vi "ReadData_9229.vi"(8 "error in":errorcluster, 11 "Module Config Selector":i16) -> (0 "error out":errorcluster, 1 "Number Of Pulses":u32, 2 "OversampleClk Ticks":u32, 3 "Data Array":sgl[](array[numeric]) format="%.2f")   [LabVIEW 2017, in "VDMS_VibAPI_8.lvlib"]
uses:
  <vilib>/addons/InsightCM/Devices/Shared/Cms/Fpga/AcquisitionFpgaTach/source/subVIs/VibAPI_8/VDMS_VibAPI_8.lvlib
  <vilib>/rvi/eio/common/nirviEmuTemplateMethod_errors.vi
  <vilib>/rvi/Memory/Memory_Emulation/nirvimemoryFastEmulation.vi
  <vilib>/rvi/Memory/Memory_Emulation/nirvimemoryEmulation.vi
  <vilib>/rvi/Emulation/niFpgaEmulationIsFPGAContextNoSignature.vi
  <vilib>/rvi/DataTransferAndStorage/Container/Common/niFpgaContainerGetUniqueNameForEmu.vi
  <vilib>/rvi/Emulation/niFpgaProcessEmulError.vi
  <vilib>/rvi/Emulation/niFpgaSctlEmulationGetInTimedLoop.vi
  <vilib>/rvi/errors/nirviReportUnexpectedCaseInternalError (U32).vi
  <vilib>/eio/EIONode/EIONode.xnode
  <vilib>/rvi/DataTransferAndStorage/Container/XNode/niFpgaContainer.xnode
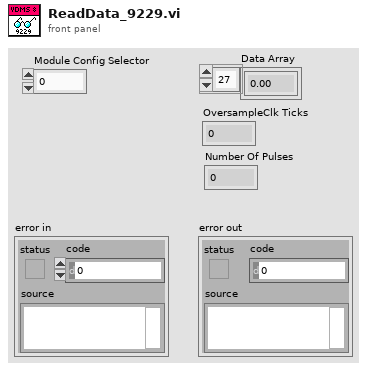
[diagram p1: front panel]
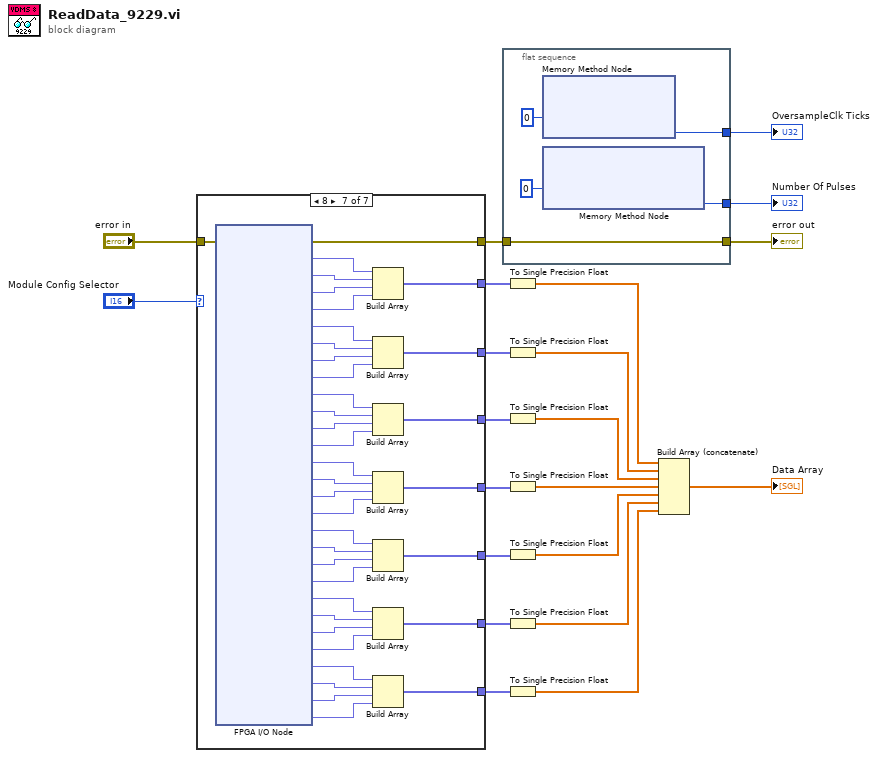
[diagram p0: block diagram]
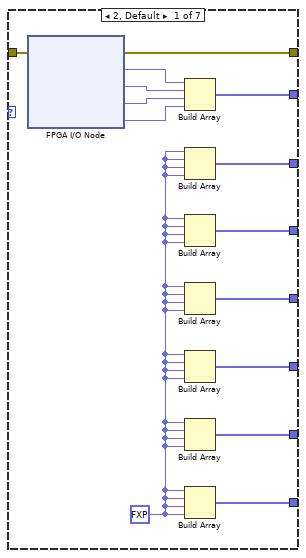
[diagram p2: hidden frame]
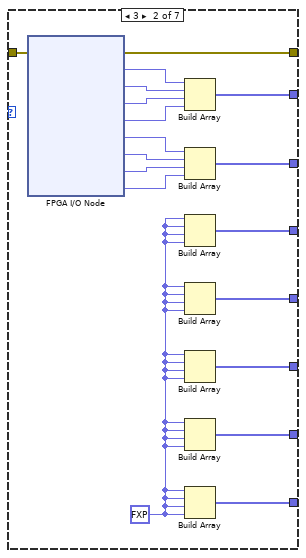
[diagram p3: hidden frame]
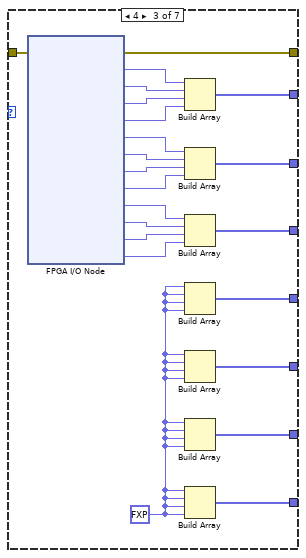
[diagram p4: hidden frame]
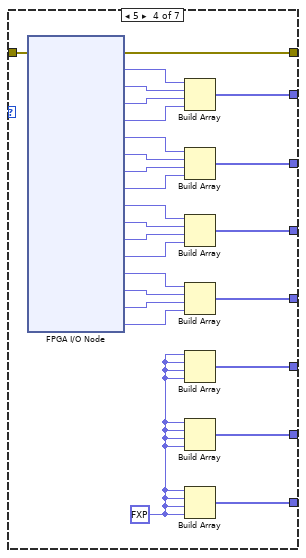
[diagram p5: hidden frame]
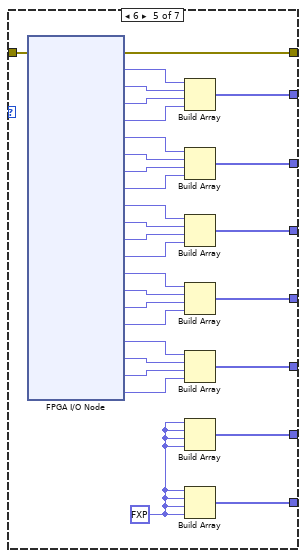
[diagram p6: hidden frame]
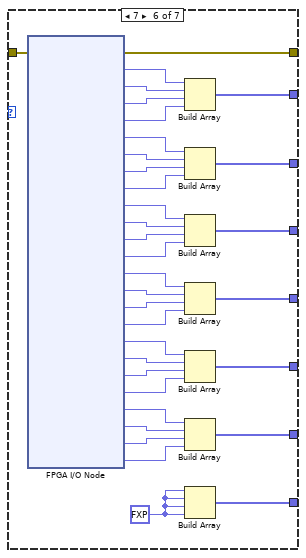
[diagram p7: hidden frame]
diagram:
  n1 = case shown="8" "Module Config Selector" {
    tunnel: "error in" -> [w35 w53 w75 w101 w131 w165 w202]
    tunnel: [w34 w52 w74 w100 w130 w164 w201] -> w21
    tunnel: [w33 w51 w73 w99 w129 w163 w200] -> w17
    tunnel: [w32 w50 w72 w98 w128 w162 w199] -> w15
    tunnel: [w31 w49 w71 w97 w127 w161 w198] -> w12
    tunnel: [w30 w48 w70 w96 w126 w160 w197] -> w10
    tunnel: [w29 w47 w69 w95 w125 w159 w196] -> w8
    tunnel: [w28 w46 w68 w94 w124 w158 w195] -> w6
    tunnel: [w27 w45 w67 w93 w123 w157 w194] -> w4
    frame 2, Default {
      w22 = fxp<+/-,24,7> 0.0 ("Mod1/AI2")
      n2 = xnode "FPGA I/O Node"("error in"=w35) -> ("error out"=w34:errorcluster, "Mod2/AI0"=w25:fxp<+/-,24,7>, "Mod2/AI1"=w26:fxp<+/-,24,7>, "Mod2/AI2"=w24:fxp<+/-,24,7>, "Mod2/AI3"=w23:fxp<+/-,24,7>)  [unwired: 4 in, 4 out]
      n3 = Build Array(w25, w26, w24, w23) -> (w33:fxp<+/-,24,7>[])
      n4 = Build Array(w22, w22, w22, w22) -> (w32:fxp<+/-,24,7>[])
      n5 = Build Array(w22, w22, w22, w22) -> (w31:fxp<+/-,24,7>[])
      n6 = Build Array(w22, w22, w22, w22) -> (w30:fxp<+/-,24,7>[])
      n7 = Build Array(w22, w22, w22, w22) -> (w29:fxp<+/-,24,7>[])
      n8 = Build Array(w22, w22, w22, w22) -> (w28:fxp<+/-,24,7>[])
      n9 = Build Array(w22, w22, w22, w22) -> (w27:fxp<+/-,24,7>[])
    }
    frame 3 {
      w36 = fxp<+/-,24,7> 0.0 ("Mod1/AI2")
      n10 = xnode "FPGA I/O Node"("error in"=w53) -> ("error out"=w52:errorcluster, "Mod2/AI0"=w41:fxp<+/-,24,7>, "Mod2/AI1"=w42:fxp<+/-,24,7>, "Mod2/AI2"=w40:fxp<+/-,24,7>, "Mod2/AI3"=w38:fxp<+/-,24,7>, "Mod3/AI0"=w39:fxp<+/-,24,7>, "Mod3/AI1"=w43:fxp<+/-,24,7>, "Mod3/AI2"=w44:fxp<+/-,24,7>, "Mod3/AI3"=w37:fxp<+/-,24,7>)  [unwired: 8 in, 8 out]
      n11 = Build Array(w41, w42, w40, w38) -> (w51:fxp<+/-,24,7>[])
      n12 = Build Array(w39, w43, w44, w37) -> (w50:fxp<+/-,24,7>[])
      n13 = Build Array(w36, w36, w36, w36) -> (w49:fxp<+/-,24,7>[])
      n14 = Build Array(w36, w36, w36, w36) -> (w48:fxp<+/-,24,7>[])
      n15 = Build Array(w36, w36, w36, w36) -> (w47:fxp<+/-,24,7>[])
      n16 = Build Array(w36, w36, w36, w36) -> (w46:fxp<+/-,24,7>[])
      n17 = Build Array(w36, w36, w36, w36) -> (w45:fxp<+/-,24,7>[])
    }
    frame 4 {
      w54 = fxp<+/-,24,7> 0.0 ("Mod1/AI2")
      n18 = xnode "FPGA I/O Node"("error in"=w75) -> ("error out"=w74:errorcluster, "Mod2/AI0"=w60:fxp<+/-,24,7>, "Mod2/AI1"=w61:fxp<+/-,24,7>, "Mod2/AI2"=w59:fxp<+/-,24,7>, "Mod2/AI3"=w57:fxp<+/-,24,7>, "Mod3/AI0"=w58:fxp<+/-,24,7>, "Mod3/AI1"=w62:fxp<+/-,24,7>, "Mod3/AI2"=w63:fxp<+/-,24,7>, "Mod3/AI3"=w56:fxp<+/-,24,7>, "Mod4/AI0"=w64:fxp<+/-,24,7>, "Mod4/AI1"=w65:fxp<+/-,24,7>, "Mod4/AI2"=w66:fxp<+/-,24,7>, "Mod4/AI3"=w55:fxp<+/-,24,7>)  [unwired: 12 in, 12 out]
      n19 = Build Array(w60, w61, w59, w57) -> (w73:fxp<+/-,24,7>[])
      n20 = Build Array(w58, w62, w63, w56) -> (w72:fxp<+/-,24,7>[])
      n21 = Build Array(w64, w65, w66, w55) -> (w71:fxp<+/-,24,7>[])
      n22 = Build Array(w54, w54, w54, w54) -> (w70:fxp<+/-,24,7>[])
      n23 = Build Array(w54, w54, w54, w54) -> (w69:fxp<+/-,24,7>[])
      n24 = Build Array(w54, w54, w54, w54) -> (w68:fxp<+/-,24,7>[])
      n25 = Build Array(w54, w54, w54, w54) -> (w67:fxp<+/-,24,7>[])
    }
    frame 5 {
      w76 = fxp<+/-,24,7> 0.0 ("Mod1/AI2")
      n26 = xnode "FPGA I/O Node"("error in"=w101) -> ("error out"=w100:errorcluster, "Mod2/AI0"=w83:fxp<+/-,24,7>, "Mod2/AI1"=w84:fxp<+/-,24,7>, "Mod2/AI2"=w82:fxp<+/-,24,7>, "Mod2/AI3"=w80:fxp<+/-,24,7>, "Mod3/AI0"=w81:fxp<+/-,24,7>, "Mod3/AI1"=w85:fxp<+/-,24,7>, "Mod3/AI2"=w86:fxp<+/-,24,7>, "Mod3/AI3"=w79:fxp<+/-,24,7>, "Mod4/AI0"=w87:fxp<+/-,24,7>, "Mod4/AI1"=w88:fxp<+/-,24,7>, "Mod4/AI2"=w89:fxp<+/-,24,7>, "Mod4/AI3"=w78:fxp<+/-,24,7>, "Mod5/AI0"=w90:fxp<+/-,24,7>, "Mod5/AI1"=w91:fxp<+/-,24,7>, "Mod5/AI2"=w92:fxp<+/-,24,7>, "Mod5/AI3"=w77:fxp<+/-,24,7>)  [unwired: 16 in, 16 out]
      n27 = Build Array(w83, w84, w82, w80) -> (w99:fxp<+/-,24,7>[])
      n28 = Build Array(w81, w85, w86, w79) -> (w98:fxp<+/-,24,7>[])
      n29 = Build Array(w87, w88, w89, w78) -> (w97:fxp<+/-,24,7>[])
      n30 = Build Array(w90, w91, w92, w77) -> (w96:fxp<+/-,24,7>[])
      n31 = Build Array(w76, w76, w76, w76) -> (w95:fxp<+/-,24,7>[])
      n32 = Build Array(w76, w76, w76, w76) -> (w94:fxp<+/-,24,7>[])
      n33 = Build Array(w76, w76, w76, w76) -> (w93:fxp<+/-,24,7>[])
    }
    frame 6 {
      w102 = fxp<+/-,24,7> 0.0 ("Mod1/AI2")
      n34 = xnode "FPGA I/O Node"("error in"=w131) -> ("error out"=w130:errorcluster, "Mod2/AI0"=w110:fxp<+/-,24,7>, "Mod2/AI1"=w111:fxp<+/-,24,7>, "Mod2/AI2"=w109:fxp<+/-,24,7>, "Mod2/AI3"=w107:fxp<+/-,24,7>, "Mod3/AI0"=w108:fxp<+/-,24,7>, "Mod3/AI1"=w112:fxp<+/-,24,7>, "Mod3/AI2"=w113:fxp<+/-,24,7>, "Mod3/AI3"=w106:fxp<+/-,24,7>, "Mod4/AI0"=w114:fxp<+/-,24,7>, "Mod4/AI1"=w115:fxp<+/-,24,7>, "Mod4/AI2"=w116:fxp<+/-,24,7>, "Mod4/AI3"=w105:fxp<+/-,24,7>, "Mod5/AI0"=w117:fxp<+/-,24,7>, "Mod5/AI1"=w118:fxp<+/-,24,7>, "Mod5/AI2"=w119:fxp<+/-,24,7>, "Mod5/AI3"=w104:fxp<+/-,24,7>, "Mod6/AI0"=w120:fxp<+/-,24,7>, "Mod6/AI1"=w121:fxp<+/-,24,7>, "Mod6/AI2"=w122:fxp<+/-,24,7>, "Mod6/AI3"=w103:fxp<+/-,24,7>)  [unwired: 20 in, 20 out]
      n35 = Build Array(w110, w111, w109, w107) -> (w129:fxp<+/-,24,7>[])
      n36 = Build Array(w108, w112, w113, w106) -> (w128:fxp<+/-,24,7>[])
      n37 = Build Array(w114, w115, w116, w105) -> (w127:fxp<+/-,24,7>[])
      n38 = Build Array(w117, w118, w119, w104) -> (w126:fxp<+/-,24,7>[])
      n39 = Build Array(w120, w121, w122, w103) -> (w125:fxp<+/-,24,7>[])
      n40 = Build Array(w102, w102, w102, w102) -> (w124:fxp<+/-,24,7>[])
      n41 = Build Array(w102, w102, w102, w102) -> (w123:fxp<+/-,24,7>[])
    }
    frame 7 {
      w132 = fxp<+/-,24,7> 0.0 ("Mod1/AI2")
      n42 = xnode "FPGA I/O Node"("error in"=w165) -> ("error out"=w164:errorcluster, "Mod2/AI0"=w144:fxp<+/-,24,7>, "Mod2/AI1"=w145:fxp<+/-,24,7>, "Mod2/AI2"=w140:fxp<+/-,24,7>, "Mod2/AI3"=w138:fxp<+/-,24,7>, "Mod3/AI0"=w139:fxp<+/-,24,7>, "Mod3/AI1"=w146:fxp<+/-,24,7>, "Mod3/AI2"=w147:fxp<+/-,24,7>, "Mod3/AI3"=w137:fxp<+/-,24,7>, "Mod4/AI0"=w148:fxp<+/-,24,7>, "Mod4/AI1"=w149:fxp<+/-,24,7>, "Mod4/AI2"=w150:fxp<+/-,24,7>, "Mod4/AI3"=w136:fxp<+/-,24,7>, "Mod5/AI0"=w151:fxp<+/-,24,7>, "Mod5/AI1"=w152:fxp<+/-,24,7>, "Mod5/AI2"=w153:fxp<+/-,24,7>, "Mod5/AI3"=w135:fxp<+/-,24,7>, "Mod6/AI0"=w154:fxp<+/-,24,7>, "Mod6/AI1"=w155:fxp<+/-,24,7>, "Mod6/AI2"=w156:fxp<+/-,24,7>, "Mod6/AI3"=w134:fxp<+/-,24,7>, "Mod7/AI0"=w143:fxp<+/-,24,7>, "Mod7/AI1"=w142:fxp<+/-,24,7>, "Mod7/AI2"=w141:fxp<+/-,24,7>, "Mod7/AI3"=w133:fxp<+/-,24,7>)  [unwired: 24 in, 24 out]
      n43 = Build Array(w144, w145, w140, w138) -> (w163:fxp<+/-,24,7>[])
      n44 = Build Array(w139, w146, w147, w137) -> (w162:fxp<+/-,24,7>[])
      n45 = Build Array(w148, w149, w150, w136) -> (w161:fxp<+/-,24,7>[])
      n46 = Build Array(w151, w152, w153, w135) -> (w160:fxp<+/-,24,7>[])
      n47 = Build Array(w154, w155, w156, w134) -> (w159:fxp<+/-,24,7>[])
      n48 = Build Array(w143, w142, w141, w133) -> (w158:fxp<+/-,24,7>[])
      n49 = Build Array(w132, w132, w132, w132) -> (w157:fxp<+/-,24,7>[])
    }
    frame 8 {
      n50 = xnode "FPGA I/O Node"("error in"=w202) -> ("error out"=w201:errorcluster, "Mod2/AI0"=w181:fxp<+/-,24,7>, "Mod2/AI1"=w182:fxp<+/-,24,7>, "Mod2/AI2"=w174:fxp<+/-,24,7>, "Mod2/AI3"=w172:fxp<+/-,24,7>, "Mod3/AI0"=w173:fxp<+/-,24,7>, "Mod3/AI1"=w183:fxp<+/-,24,7>, "Mod3/AI2"=w184:fxp<+/-,24,7>, "Mod3/AI3"=w171:fxp<+/-,24,7>, "Mod4/AI0"=w185:fxp<+/-,24,7>, "Mod4/AI1"=w186:fxp<+/-,24,7>, "Mod4/AI2"=w187:fxp<+/-,24,7>, "Mod4/AI3"=w170:fxp<+/-,24,7>, "Mod5/AI0"=w188:fxp<+/-,24,7>, "Mod5/AI1"=w189:fxp<+/-,24,7>, "Mod5/AI2"=w190:fxp<+/-,24,7>, "Mod5/AI3"=w169:fxp<+/-,24,7>, "Mod6/AI0"=w191:fxp<+/-,24,7>, "Mod6/AI1"=w192:fxp<+/-,24,7>, "Mod6/AI2"=w193:fxp<+/-,24,7>, "Mod6/AI3"=w168:fxp<+/-,24,7>, "Mod7/AI0"=w180:fxp<+/-,24,7>, "Mod7/AI1"=w179:fxp<+/-,24,7>, "Mod7/AI2"=w178:fxp<+/-,24,7>, "Mod7/AI3"=w166:fxp<+/-,24,7>, "Mod8/AI0"=w177:fxp<+/-,24,7>, "Mod8/AI1"=w176:fxp<+/-,24,7>, "Mod8/AI2"=w175:fxp<+/-,24,7>, "Mod8/AI3"=w167:fxp<+/-,24,7>)  [unwired: 28 in, 28 out]
      n51 = Build Array(w181, w182, w174, w172) -> (w200:fxp<+/-,24,7>[])
      n52 = Build Array(w173, w183, w184, w171) -> (w199:fxp<+/-,24,7>[])
      n53 = Build Array(w185, w186, w187, w170) -> (w198:fxp<+/-,24,7>[])
      n54 = Build Array(w188, w189, w190, w169) -> (w197:fxp<+/-,24,7>[])
      n55 = Build Array(w191, w192, w193, w168) -> (w196:fxp<+/-,24,7>[])
      n56 = Build Array(w180, w179, w178, w166) -> (w195:fxp<+/-,24,7>[])
      n57 = Build Array(w177, w176, w175, w167) -> (w194:fxp<+/-,24,7>[])
    }
  }
  n58 = flat-sequence {
    tunnel: w21 -> [w207]
    tunnel: [w207] -> w20
    tunnel: [w206] -> w19
    tunnel: [w203] -> w18
    frame #0 {
      n59 = xnode ("Memory Method Node")("Address"=u32 0) -> ("Data"=w206:u32)  [unwired: 1 in, 1 out]
      n60 = xnode ("Memory Method Node")("Address"=u32 0) -> ("Data"=w203:u32)  [unwired: 1 in, 1 out]
    }
  }
  n61 = To Single Precision Float(number=w17) -> (single precision float=w16:sgl[])
  n62 = To Single Precision Float(number=w15) -> (single precision float=w14:sgl[])
  n63 = To Single Precision Float(number=w12) -> (single precision float=w11:sgl[])
  n64 = To Single Precision Float(number=w10) -> (single precision float=w9:sgl[])
  n65 = To Single Precision Float(number=w8) -> (single precision float=w7:sgl[])
  n66 = To Single Precision Float(number=w6) -> (single precision float=w5:sgl[])
  n67 = To Single Precision Float(number=w4) -> (single precision float=w3:sgl[])
  n68 = Build Array (concatenate)(w16, w14, w11, w9, w7, w5, w3) -> (→"Data Array":sgl[])
  "error out" <- w20
  "OversampleClk Ticks" <- w19
  "Number Of Pulses" <- w18
